vi "Get images.vi"() -> ()   [LabVIEW 2014]
uses:
  <vilib>/zip/NI_Unzip.lvlib
  <vilib>/ErrorRing/Error Ring.xnode
  <vilib>/Utility/error.llb/Error Cluster From Error Code.vi
panel:
  out "error out":errorcluster
  out "Images":picture[](array[picture])
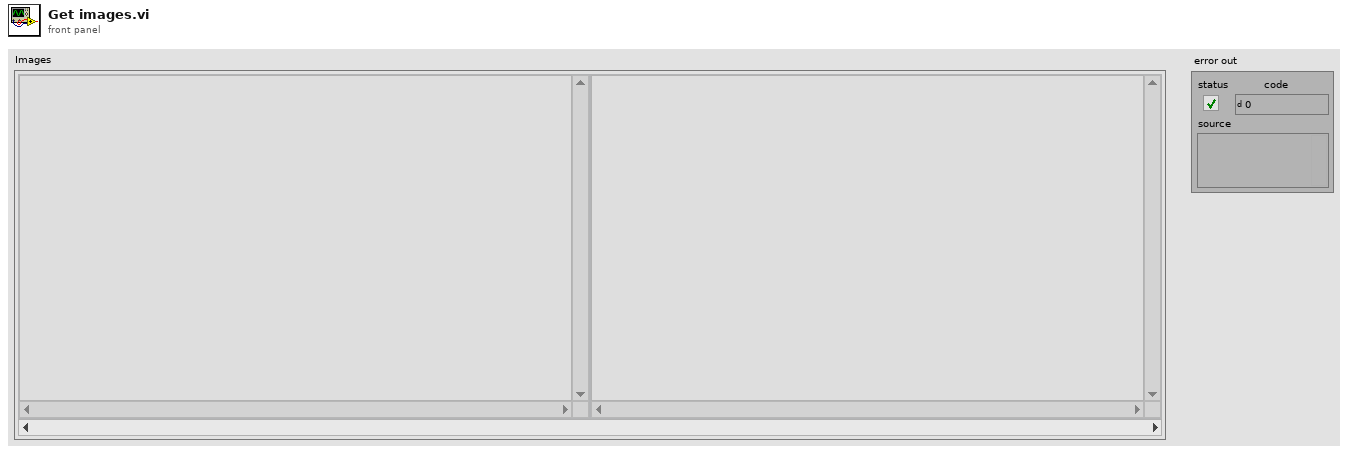
[diagram p1: front panel]
types:
  T1 = cluster{"left":i16, "top":i16, "right":i16, "bottom":i16}
  T2 = typedef "imagedata.ctl" = cluster{"image type":i32, "image depth":i32, "image":u8[], "mask":u8[], "colors":u32[], "Rectangle":cluster{"left":i16, "top":i16, "right":i16, "bottom":i16}}
  T3 = typedef "LVBoundsTypeDef.ctl" = cluster{"Width":u32, "Height":u32}
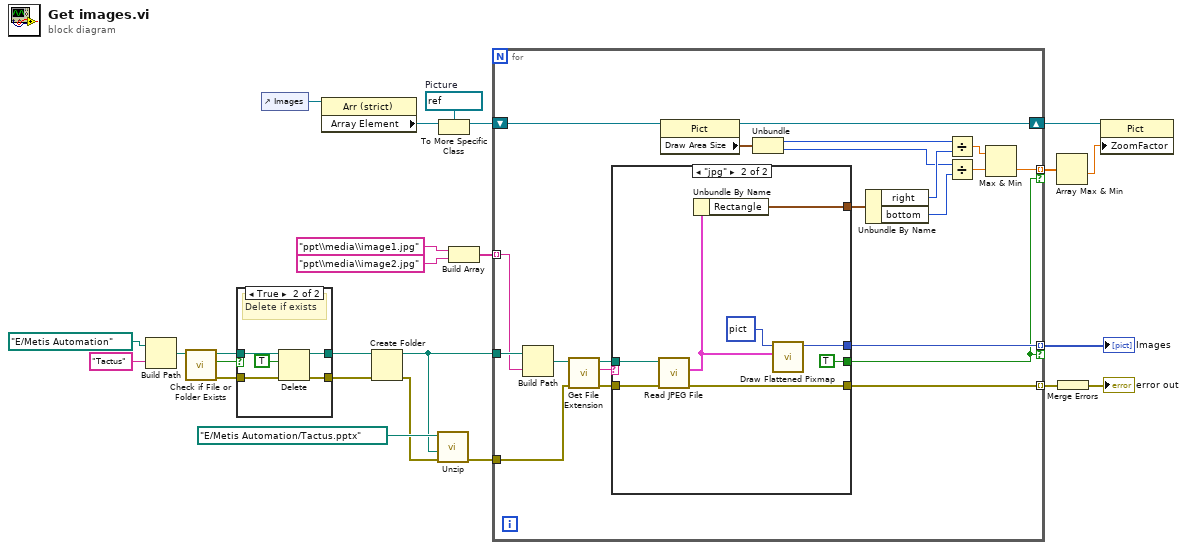
[diagram p0: block diagram]
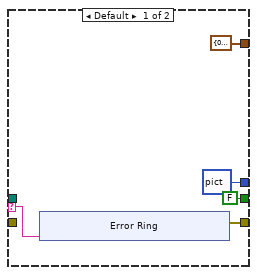
[diagram p2: hidden frame]
diagram:
  w5 = refnum<vi> refnum  # Picture
  n1 = Build Path(base path=path "E:/Metis Automation", name or relative path="Tactus") -> (appended path=w23:path)
  n2 = call <vilib>:"Check if File or Folder Exists.vi"("path"=w23) -> ("error out"=w20:errorcluster, "file or folder exists?"=w21:bool, "dup path"=w22:path)  [unwired: 8 in]
  n3 = case shown="True" w21 {
    tunnel: w22 -> [w26 w32]
    tunnel: w20 -> [w27 w31]
    tunnel: [w27 w30] -> w18
    tunnel: [w26 w29] -> w19
    frame False {
    }
    frame True {
      # "Delete if exists"
      n4 = Delete(path (use dialog)=w32, entire hierarchy (F)=TRUE, error in=w31) -> (deleted path=w29:path, error out=w30:errorcluster)  [unwired: 2 in, 1 out]
    }
  }
  n5 = control-ref of="Images"() -> (w7:refnum<vi>)
  n6 = property class="Arr (strict)"(reference=w7) -> ("Array Element"=w6:refnum<vi>)  [unwired: 1 in, 2 out]
  n7 = Create Folder(path (use dialog)=w19, error in=w18) -> (created path=w16:path, error out=w15:errorcluster)  [unwired: 1 in, 1 out]
  n8 = call <vilib>:"Unzip.vi"("error in (no error)"=w15, "Target directory (same as Zip file if empty)"=w16, "Zip file"=path "E:/Metis Automation/Tactus.pptx") -> ("error out"=w14:errorcluster)  [unwired: 6 in, 2 out]
  n9 = To More Specific Class(target class=w5, reference=w6) -> (specific class reference=w4:refnum<vi>)  [unwired: 1 in, 1 out]
  n10 = Build Array("ppt\\media\\image1.jpg", "ppt\\media\\image2.jpg") -> (w11:string[])
  n11 = for {
    tunnel: w16 -> [w53]
    tunnel: w14 -> [w48]
    tunnel: w11 -> [w52] mode=indexing
    tunnel: [w46] -> w10 mode=indexing if=w35
    tunnel: [w45] -> w9 mode=indexing
    tunnel: [w34] -> w2 mode=indexing if=w35
    shift-right: [w33] -> w3
    shift-left: w4 -> [w43]
    n12 = Build Path(base path=w53, name or relative path=w52) -> (appended path=w51:path)
    n13 = call <vilib>:"Get File Extension.vi"("error in (no error)"=w48, "file"=w51) -> ("error out"=w47:errorcluster, "lowercase file extension"=w49:string, "dup file"=w50:path)  [unwired: 5 in, 2 out]
    n14 = case shown="\"jpg\"" w49 {
      selector: w49 -> [w58 _]
      tunnel: w50 -> [_ w73]
      tunnel: w47 -> [_ w72]
      tunnel: [w57 w68] -> w45
      tunnel: [picture data[5B] ("new picture") w70] -> w46
      tunnel: [FALSE TRUE] -> w35
      tunnel: [T1 {"left"=0, "top"=0, "right"=0, "bottom"=0} ("Rectangle") w66] -> w41
      frame Default {
        n15 = xnode "Error Ring"("parameter 0"=w58) -> ("error out"=w57:errorcluster)
      }
      frame "jpg" {
        n16 = call <vilib>:"Read JPEG File.vi"("error in (no error)"=w72, "path to JPEG file"=w73) -> ("error out"=w68:errorcluster, "image data"=w67:T2)  [unwired: 7 in, 1 out]
        n17 = Unbundle By Name(w67) -> ("Rectangle"=w66:T1)
        n18 = call <vilib>:"Draw Flattened Pixmap.vi"("image data"=w67, "picture"=picture data[5B]) -> ("new picture"=w70:picture)  [unwired: 7 in]
      }
    }
    n19 = property class="Pict"(reference=w43) -> (reference out=w33:refnum<vi>, "Draw Area Size"=w44:T3)  [unwired: 1 in, 1 out]
    n20 = Unbundle(w44) -> ("Width"=w42:u32, "Height"=w39:u32)
    n21 = Unbundle By Name(w41) -> ("right"=w40:i16, "bottom"=w38:i16)
    n22 = Divide(x=w42, y=w40) -> (x/y=w37:dbl)
    n23 = Divide(x=w39, y=w38) -> (x/y=w36:dbl)
    n24 = Max & Min(x=w37, y=w36) -> (min(x,y)=w34:dbl)  [unwired: 1 out]
  }
  "Images" <- w10
  n25 = Array Max & Min(array=w2) -> (min value=w1:dbl)  [unwired: 3 out]
  n26 = Merge Errors(w9) -> (→"error out":errorcluster)
  n27 = property class="Pict"(reference=w3, "ZoomFactor"=w1) -> ()  [unwired: 1 in, 2 out]
